vi "Update Global.vi"(10 "Val":cluster{"Complexity":u64, "Current":string}, 11 "Key":T1) -> ()   [LabVIEW 2020]
uses:
  Memory Global.vi
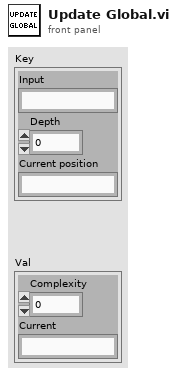
[diagram p1: front panel]
types:
  T1 = cluster{"Input":string, "Depth":u32, "Current position":string}
  T2 = map{cluster{"Input":string, "Depth":u32, "Current position":string}, cluster{"default value":u64, "default value":string}}
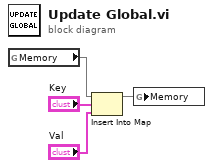
[diagram p0: block diagram]
diagram:
  n1 = global read "Memory Global.vi" "Memory"() -> (w1:T2)
  n2 = Insert Into Map(map in=w1, key="Key", value="Val") -> (map out=w2:T2)  [unwired: 2 out]
  n3 = global write "Memory Global.vi" "Memory"(w2) -> ()
